vi "FlushSerialBuffer.vi"(2 "error in (no error)":errorcluster, 3 "VISA resource name":refnum<visa-resource-name>="COM8") -> (0 "error out":errorcluster, 1 "VISA resource out":refnum<visa-resource-name>)   [LabVIEW 2012]
panel:
  out "return count":u32
  out "read buffer":string
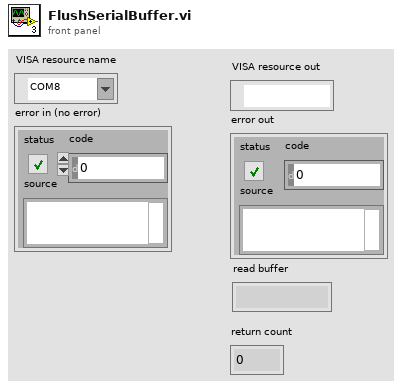
[diagram p1: front panel]
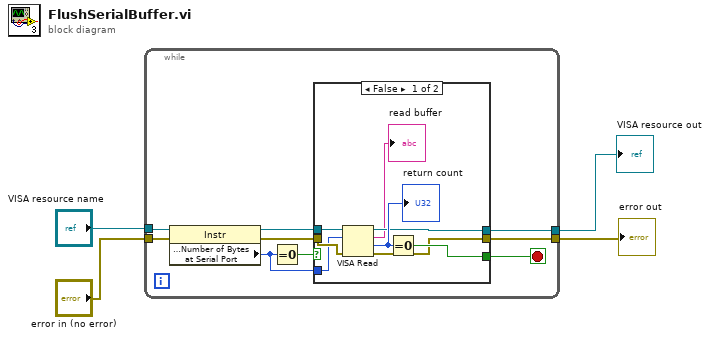
[diagram p0: block diagram]
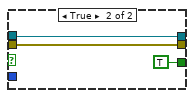
[diagram p2: hidden frame]
diagram:
  n1 = while {
    tunnel: [w12] -> w1
    tunnel: [w11] -> w2
    tunnel: "VISA resource name" -> [w10]
    tunnel: "error in (no error)" -> [w9]
    stop <- w13 stop-if-true
    n2 = property class="Instr"(reference=w10, error in=w9) -> (reference out=w7:refnum<visa-resource-name>, error out=w6:errorcluster, "Serial Settings:Number of Bytes at Serial Port"=w5:u32)
    n3 = Equal To 0?(x=w5) -> (x = 0?=w8:bool)
    n4 = case shown="False" w8 {
      tunnel: [w20 TRUE] -> w13
      tunnel: [w19 w23] -> w12
      tunnel: [w18 w24] -> w11
      tunnel: w7 -> [w16 w24]
      tunnel: w6 -> [w15 w23]
      tunnel: w5 -> [w14 _]
      frame False {
        n5 = VISA Read(VISA resource name=w16, byte count=w14, error in (no error)=w15) -> (VISA resource name out=w18:refnum<visa-resource-name>, read buffer=→"read buffer":string, return count=w21:u32, error out=w19:errorcluster)
        "return count" <- w21
        n6 = Equal To 0?(x=w21) -> (x = 0?=w20:bool)
      }
      frame True {
      }
    }
  }
  "VISA resource out" <- w2
  "error out" <- w1
